vi "Parse and Remove Lines for Downlink.vi"(10 "Input String":string) -> (2 "Output String":string)   [LabVIEW 2010]
doc: "This VI removes all blank lines and all lines that begin with \"-- PULSE\" from the input string and outputs the resulting string to the Output String indicator."
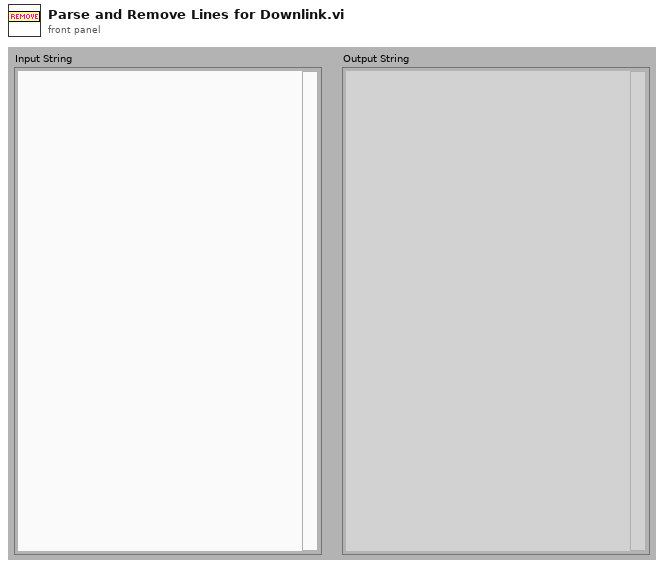
[diagram p1: front panel]
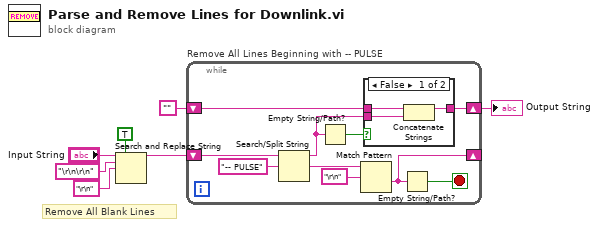
[diagram p0: block diagram]
diagram:
  # "Remove All Blank Lines"
  n1 = Search and Replace String(replace all?=TRUE ("replace all? (F)"), input string="Input String", search string="\r\n\r\n", replace string="\r\n" ("search string")) -> (result string=w5:string)  [unwired: 4 in, 3 out]
  n2 = while "Remove All Lines Beginning with -- PULSE" {
    shift-right: [w17] -> w7
    shift-left: "" -> [w16]
    shift-right: [w10] -> _
    shift-left: w5 -> [w9]
    stop <- w15 stop-if-true
    n3 = Search/Split String(string=w9, search string/char (-)="-- PULSE") -> (substring before match=w11:string, match + rest of string=w14:string)  [unwired: 1 in, 1 out]
    n4 = Empty String/Path?(string/path=w11) -> (empty?=w12:bool)
    n5 = Match Pattern(string=w14, regular expression="\r\n" ("search string/char (-)")) -> (after substring=w10:string)  [unwired: 1 in, 3 out]
    n6 = case shown="False" w12 {
      tunnel: [w20 w21] -> w17
      tunnel: w16 -> [w19 w21]
      tunnel: w11 -> [w18 _]
      frame False {
        n7 = Concatenate Strings(w19, w18) -> (w20:string)
      }
      frame True {
      }
    }
    n8 = Empty String/Path?(string/path=w10) -> (empty?=w15:bool)
  }
  "Output String" <- w7
